vi "Parse Auto Data.vi"(10 "Is Blue Alliance?":bool=TRUE, 11 "path":path) -> (0 "dt array":dbl[](array[numeric]), 1 "Zero Velocity?":bool[](array[boolean]), 2 "Velocities":T3[](array[typedef]), 3 "Positions":cluster{"x":dbl, "y":dbl, "th":dbl}[](array[cluster]), 5 "Commands out":cluster{"Time (s)":dbl, T1, bool}[](array[cluster]), 7 "Overall":cluster{"Time (s)":dbl, "Distance (ft)":dbl})   [LabVIEW 2025]
uses:
  swerve-template/Type Definitions/Data/Robot Velocities.ctl
  bordeaux-2687-rebuilt/Bordeaux/Types/Single Cmd Info.ctl
  <vilib>/picture/picture.llb/imagedata.ctl
  <vilib>/Analysis/coordinate.llb/Angle Range (Degree).ctl
  <vilib>/Analysis/coordinate.llb/Angle Units.ctl
  <vilib>/Analysis/coordinate.llb/2D Cartesian Coordinate Rotation (Scalar).vi
  <vilib>/Analysis/coordinate.llb/Wrap Angle (scalar).vi
  <vilib>/Analysis/NI_AALPro.lvlib
  <vilib>/Analysis/NI_AAL_Angle.lvlib
panel:
  out "XY Graph":cluster{dbl[], dbl[]}[](graph)
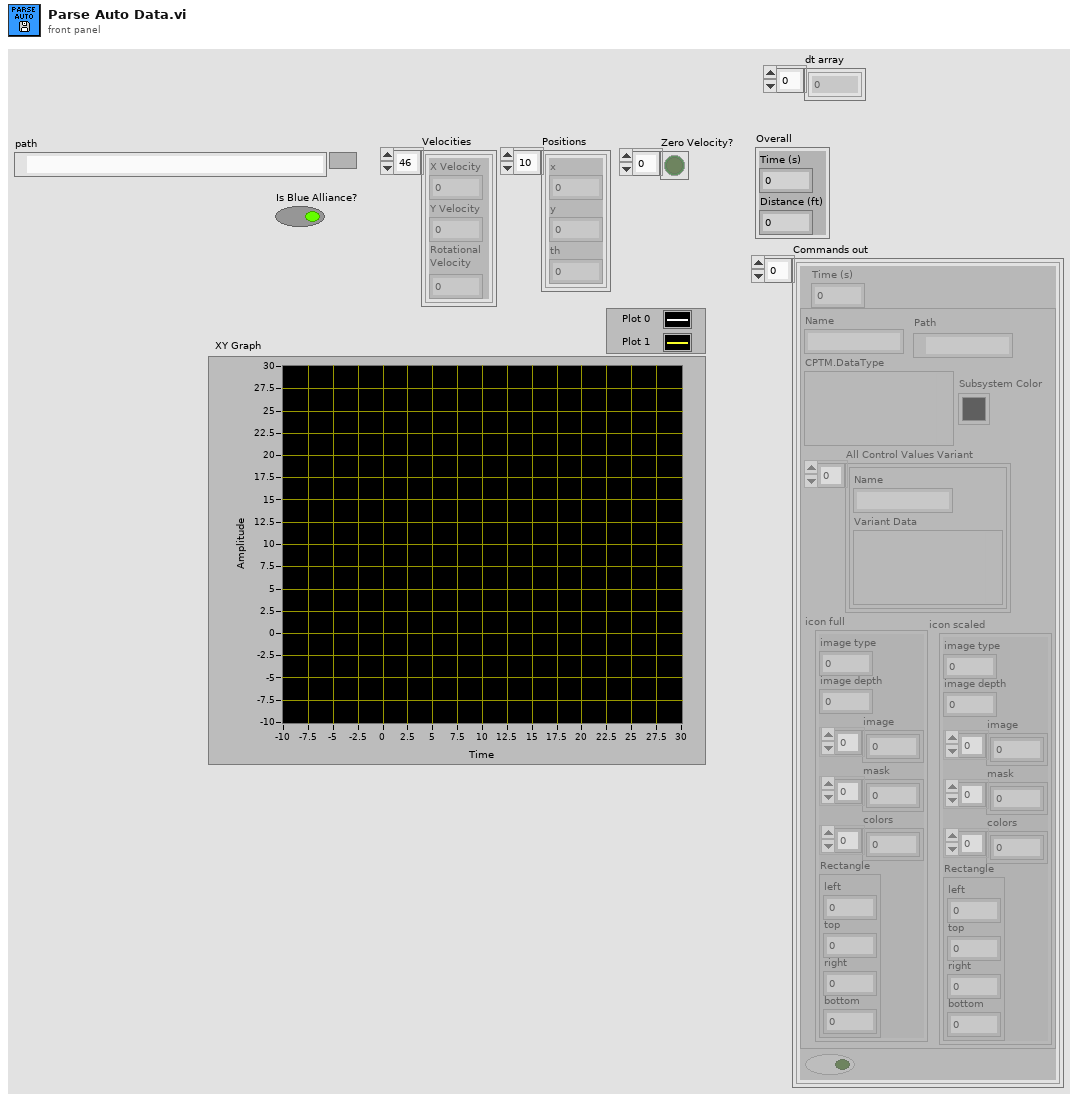
[diagram p1: front panel]
types:
  T1 = typedef "Single Cmd Info.ctl" = cluster{"Name":string, "CPTM.DataType":variant, "All Control Values Variant":cluster{"Name":string, "Variant Data":variant}[], "icon full":T2, "icon scaled":T2, "Path":path, "Subsystem Color":u32}
  T2 = typedef "imagedata.ctl" = cluster{"image type":i32, "image depth":i32, "image":u8[], "mask":u8[], "colors":u32[], "Rectangle":cluster{"left":i16, "top":i16, "right":i16, "bottom":i16}}
  T3 = typedef "Robot Velocities.ctl" = cluster{"X Velocity":dbl, "Y Velocity":dbl, "Rotational \nVelocity":dbl}
  T4 = typedef "Segment Type.ctl" = enum16{"Accel Straight", "Const Straight", "Blend", "Circle", "Bezier", "Choreo"}
  T5 = cluster{"Segment Name":string, "Type":T4, "Traj Pos Points":cluster{"x":dbl, "y":dbl, "th":dbl}[], "Traj Vel Points":cluster{"V":dbl, "Omega":dbl, "V vector":cluster{"y":dbl, "x":dbl}}[], "Accel Index":i32, "Decel Index":i32}[]
  T6 = typedef "WPI_DriverStationAllianceInfo.ctl" = enum16{"Red", "Blue", "Invalid"}
  T7 = cluster{"V":dbl, "Omega":dbl, "V vector":cluster{"y":dbl, "x":dbl}}[]
  T8 = typedef "NI_AAL_Angle.lvlib/Angle Units.ctl" = i32
  T9 = typedef "NI_AAL_Angle.lvlib/Angle Range (Degree).ctl" = u16
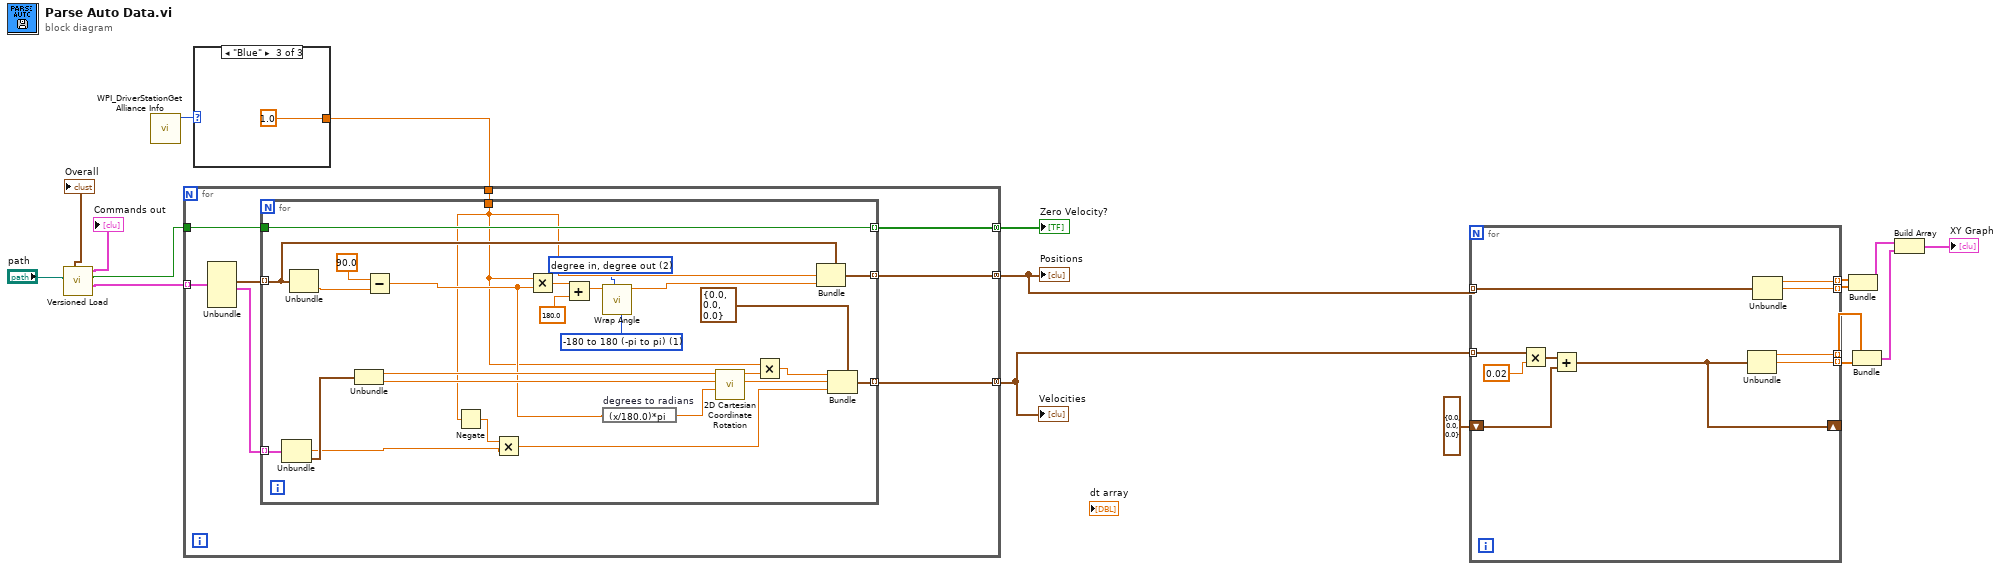
[diagram p0: block diagram]
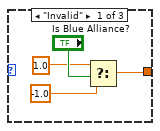
[diagram p2: hidden frame]
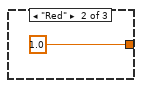
[diagram p3: hidden frame]
diagram:
  n1 = call "Versioned Load.vi"("path"="path") -> ("Trajectory Data"=w1:T5, "Zero V"=w2:bool, "Commands out"=→"Commands out":cluster{"Time (s)":dbl, T1, bool}[], "Overall"=→"Overall":cluster{"Time (s)":dbl, "Distance (ft)":dbl})  [unwired: 3 in, 4 out]
  n2 = call <vilib>:"WPI_DriverStationGet Alliance Info.vi"() -> ("Alliance"=w18:T6)  [unwired: 6 in, 5 out]
  n3 = case shown="\"Blue\"" w18 {
    tunnel: [w19 1.0 1.0] -> w17
    frame "Invalid" {
      n4 = Select(t=1.0, s="Is Blue Alliance?", f=-1.0) -> (s? t:f=w19:dbl)
    }
    frame "Red" {
    }
    frame "Blue" {
    }
  }
  n5 = for {
    tunnel: w1 -> [w32] mode=indexing
    tunnel: [w29] -> w15 mode=concatenating
    tunnel: w17 -> [w28]
    tunnel: [w25] -> w14 mode=concatenating
    tunnel: w2 -> [w27]
    tunnel: [w26] -> w16 mode=concatenating
    n6 = Unbundle(w32) -> ("Traj Pos Points"=w31:cluster{"x":dbl, "y":dbl, "th":dbl}[], "Traj Vel Points"=w30:T7)  [unwired: 4 out]
    n7 = for {
      tunnel: w31 -> [w58] mode=indexing
      tunnel: w30 -> [w56] mode=indexing
      tunnel: [w57] -> w29 mode=indexing
      tunnel: w28 -> [w39]
      tunnel: [w49] -> w25 mode=indexing
      tunnel: w27 -> [w47]
      tunnel: [w47] -> w26 mode=indexing
      w34 = T8 2 items=["radian in, radian out", "radian in, degree out", "degree in, degree out", "degree in, radian out"] ("angle units")
      w35 = T9 1 items=["none", "-180 to 180 (-pi to pi)", "0 to 360 (0 to 2pi)"] ("angle range")
      n8 = Unbundle(w56) -> ("Omega"=w41:dbl, "V vector"=w55:cluster{"y":dbl, "x":dbl})  [unwired: 1 out]
      n9 = Unbundle(w58) -> ("th"=w43:dbl)  [unwired: 2 out]
      n10 = Unbundle(w55) -> ("y"=w53:dbl, "x"=w46:dbl)
      n11 = Subtract(x=90.0, y=w43) -> (x-y=w42:dbl)
      n12 = Negate(x=w39) -> (-x=w40:dbl)
      n13 = Multiply(x=w40, y=w41) -> (x*y=w51:dbl)
      n14 = Multiply(x=w39, y=w42) -> (x*y=w38:dbl)
      n15 = Add(x=w38, y=180.0) -> (x+y=w36:dbl)
      n16 = call-poly <vilib>:"Wrap Angle.vi"("angle units"=w34, "angle range"=w35, "angle in"=w36) -> ("angle out"=w33:dbl)  [unwired: 7 in, 1 out]
      n17 = expression code="(x/180.0)*pi" "degrees to radians"(w42) -> (w54:dbl)
      n18 = call-poly <vilib>:"2D Cartesian Coordinate Rotation.vi"("theta"=w54, "y"=w46, "x"=w53) -> ("y out"=w52:dbl, "x out"=w48:dbl)  [unwired: 6 in, 1 out]
      n19 = Multiply(x=w39, y=w48) -> (x*y=w45:dbl)
      n20 = Bundle(cluster=w58, "y"=w39, "th"=w33) -> (w57:cluster{"x":dbl, "y":dbl, "th":dbl})  [unwired: 1 in]
      n21 = Bundle(cluster=T3 {"X Velocity"=0.0, "Y Velocity"=0.0, "Rotational \nVelocity"=0.0} ("Robot Velocities"), "X Velocity"=w45, "Y Velocity"=w52, "Rotational \nVelocity"=w51) -> (w49:T3)
    }
  }
  "Positions" <- w15
  "Velocities" <- w14
  "Zero Velocity?" <- w16
  n22 = for {
    tunnel: w15 -> [w68] mode=indexing
    tunnel: w14 -> [w65] mode=indexing
    tunnel: [w67] -> w13 mode=indexing
    tunnel: [w66] -> w12 mode=indexing
    shift-right: [w61] -> _
    shift-left: T3 {"X Velocity"=0.0, "Y Velocity"=0.0, "Rotational \nVelocity"=0.0} ("Robot Velocities") -> [w62]
    tunnel: [w60] -> w10 mode=indexing
    tunnel: [w59] -> w9 mode=indexing
    n23 = Multiply(x=w65, y=0.02) -> (x*y=w63:T3)
    n24 = Add(x=w63, y=w62) -> (x+y=w61:T3)
    n25 = Unbundle(w61) -> ("X Velocity"=w60:dbl, "Y Velocity"=w59:dbl)  [unwired: 1 out]
    n26 = Unbundle(w68) -> ("x"=w67:dbl, "y"=w66:dbl)  [unwired: 1 out]
  }
  n27 = Bundle(w13, w12) -> (w8:cluster{dbl[], dbl[]})  [unwired: 1 in]
  n28 = Bundle(w10, w9) -> (w7:cluster{dbl[], dbl[]})  [unwired: 1 in]
  n29 = Build Array(w8, w7) -> (→"XY Graph":cluster{dbl[], dbl[]}[])
